vi "libssh2_keepalive_send.vi"(8 "error in (no error)":errorcluster, 11 "session":T1) -> (0 "error out":errorcluster, 2 "seconds to next":i32)   [LabVIEW 2013, in "libssh2.lvlib"]
doc: "Send a keep-alive message if needed.\n\n<B>seconds to next</B> indicates how many seconds the caller can sleep before the next keep-alive message is due."
uses:
  libssh2.lvlib
  Session Refnum.ctl
  Not A Session.vi
  <vilib>/Utility/error.llb/Error Cluster From Error Code.vi
  Global Settings.vi
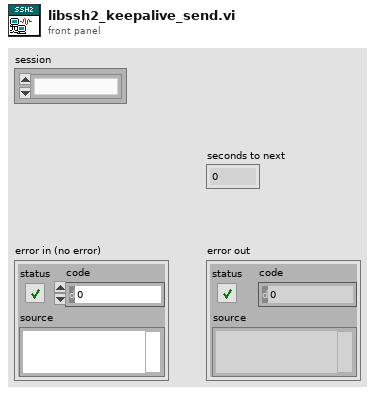
[diagram p1: front panel]
types:
  T1 = typedef "libssh2.lvlib/Session Refnum.ctl" = refnum<k1>
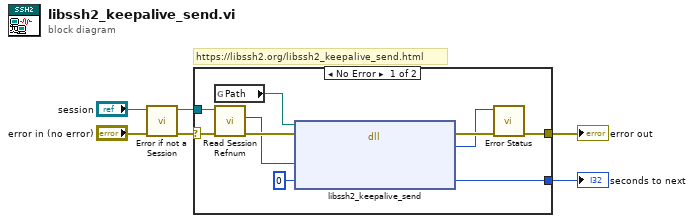
[diagram p0: block diagram]
diagram:
  # "https://libssh2.org/libssh2_keepalive_send.html"
  n1 = call "Error if not a Session.vi"("error in (no error)"="error in (no error)", "session"="session") -> ("error out"=w4:errorcluster, "session out"=w2:T1)  [unwired: 8 in]
  n2 = case shown="No Error" w4 {
    selector: w4 -> [w15 w17]
    tunnel: [w9 w17] -> w6
    tunnel: w2 -> [w14 _]
    tunnel: [w10 _] -> w1
    frame No Error {
      n3 = global read "Global Settings.vi" "Path"() -> (w11:path)
      n4 = call "Read Session Refnum.vi"("error in (no error)"=w15, "session"=w14) -> ("error out"=w13:errorcluster, "LIBSSH2_SESSION*"=w12:u64)  [unwired: 5 in, 3 out]
      n5 = dll-call lib="?" fn="libssh2_keepalive_send"(path in=w11, error in=w13, "session"=w12, "seconds_to_next"=0) -> (error out=w16:errorcluster, "return value"=w8:i32, "seconds_to_next"=w10:i32)  [unwired: 2 in, 1 out]
      n6 = call "Error Status.vi"("error in (no error)"=w16, "return value"=w8) -> ("error out"=w9:errorcluster)  [unwired: 8 in, 1 out]
    }
    frame Error {
    }
  }
  "error out" <- w6
  "seconds to next" <- w1
